vi "AddPassed_PassedIconSet.vi"() -> (0 "error out":errorcluster)   [LabVIEW 2017, in "ResultTreeListener.Tests.lvlib"]
uses:
  ResultTreeListener.Tests.lvlib
  ResultTree/Icon.ctl
  275d98eb-69a7-4435-8809-2af3ffd1cf1d.vi
  Support/FakeTestCase/FakeTestCase.lvclass
  C:/Users/de200256/Code/logmanoriginal/lvunit/Test/Test.lvclass
  Constraint/IsEqual/Create.vi
  ResultTreeListener/ResultTreeListener.lvclass
  Constraint/IsEqual/IsEqual.lvclass
  ResultTree/ResultTree.lvclass
panel:
  in  "Tree":string(tree)
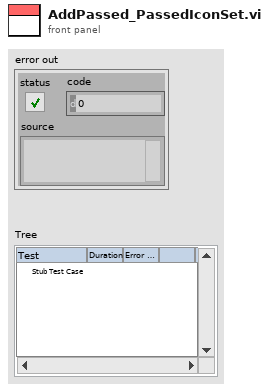
[diagram p1: front panel]
types:
  T1 = typedef "ResultTree.lvclass/Icon.ctl" = enum16{"None", "Passed", "Failed", "Error"}
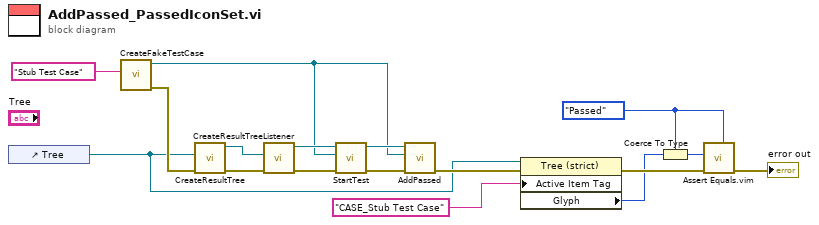
[diagram p0: block diagram]
diagram:
  w1 = Icon."Passed" ("Active Cell:String")
  n1 = control-ref of="Tree"() -> (w5:refnum<vi>)
  n2 = call "CreateFakeTestCase.vi"("Name"="Stub Test Case") -> ("error out"=w9:errorcluster, "FakeTestCase out"=w7:refnum<class "FakeTestCase.lvclass">)  [unwired: 9 in]
  n3 = call "CreateResultTree.vi"("error in (no error)"=w9, "Tree Refnum"=w5) -> ("error out"=w17:errorcluster, "ResultTree out"=w16:refnum<class "ResultTree.lvclass">)  [unwired: 8 in]
  n4 = call "CreateResultTreeListener.vi"("error in (no error)"=w17, "ResultTree"=w16) -> ("error out"=w15:errorcluster, "ResultTreeListener out"=w13:refnum<class "ResultTreeListener.lvclass">)  [unwired: 8 in]
  n5 = call-dynamic "StartTest.vi"("error in (no error)"=w15, "Test"=w7, "ResultTreeListener in"=w13) -> ("error out"=w11:errorcluster, "ResultTreeListener out"=w10:refnum<class "ResultTreeListener.lvclass">)  [unwired: 7 in]
  n6 = call-dynamic "AddPassed.vi"("error in (no error)"=w11, "Test"=w7, "ResultTreeListener in"=w10) -> ("error out"=w8:errorcluster)  [unwired: 7 in, 1 out]
  n7 = property class="Tree (strict)"(reference=w5, error in=w8, "Active Item Tag"="CASE_Stub Test Case" ("Active Item:Tag")) -> (error out=w6:errorcluster, "Glyph"=w3:i32)  [unwired: 1 out]
  n8 = Coerce To Type(0:w3, 1:w1) -> (2:w2:T1)
  n9 = call "Assert Equals.vim"("Expected"=w1, "error in (no error)"=w6, "Actual"=w2) -> ("error out"=→"error out":errorcluster)  [unwired: 8 in]
